vi "VISA Connection Write.vi"   [LabVIEW 2014, in "VISA Connection Template.lvlib"]
uses:
  VISA Connection Template.lvlib
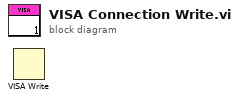
[diagram p0: block diagram]
diagram:
  n1 = VISA Write() -> ()  [unwired: 3 in, 3 out]
